vi "SCTL Period.vi"() -> (8 "Clock Period(micro second)":dbl)   [LabVIEW 2016]
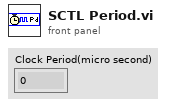
[diagram p1: front panel]
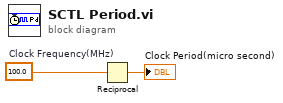
[diagram p0: block diagram]
diagram:
  w2 = 100.0  # Clock Frequency(MHz)
  n1 = Reciprocal(x=w2) -> (1/x=→"Clock Period(micro second)":dbl)
